vi "Lock In Time Trace.vi"() -> ()   [LabVIEW 2011]
panel:
  in  "VISA session (for class)":refnum<visa-resource-name>
  in  "Display Type":u16(ring) items=["X %", "Y %", "X Calibrated", "Y Calibrated", "Mag %", "Mag Calibrated", "Phase Degrees", "Ratio", "Log Ratio", "ADC 1", "ADC 2", "ADC 3", "ADC 4", "Noise %", "Noise Calibrated", "Ref Frequency", "Equation 1", "Equation 2"]
  out "XY Graph":cluster{"Y":dbl[], "Y":dbl[]}[](graph)
  in  "Time Target (s)":dbl=1.0
  in  "stop":bool
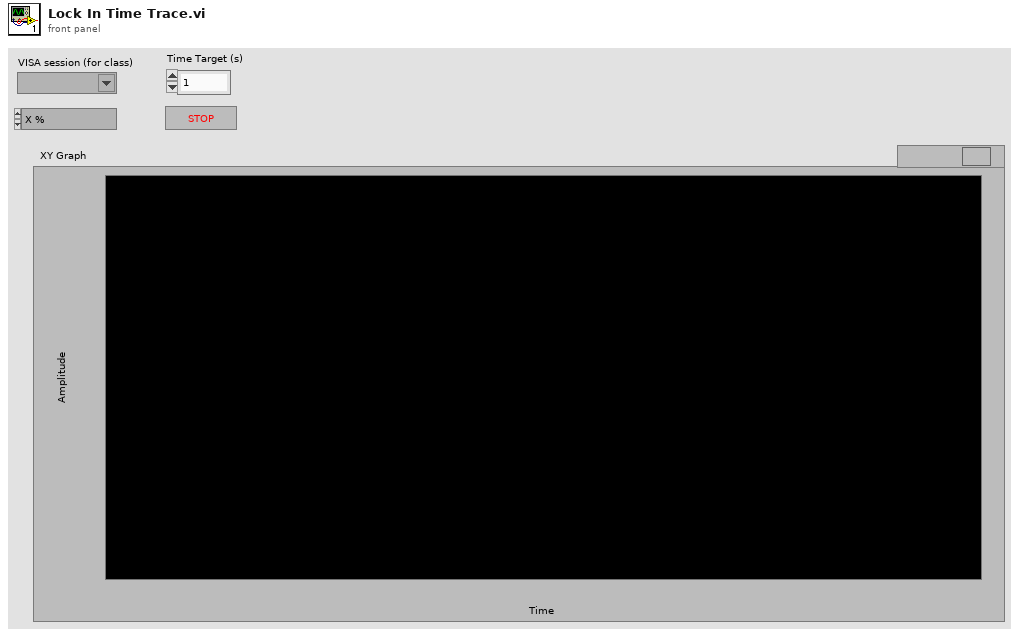
[diagram p1: front panel]
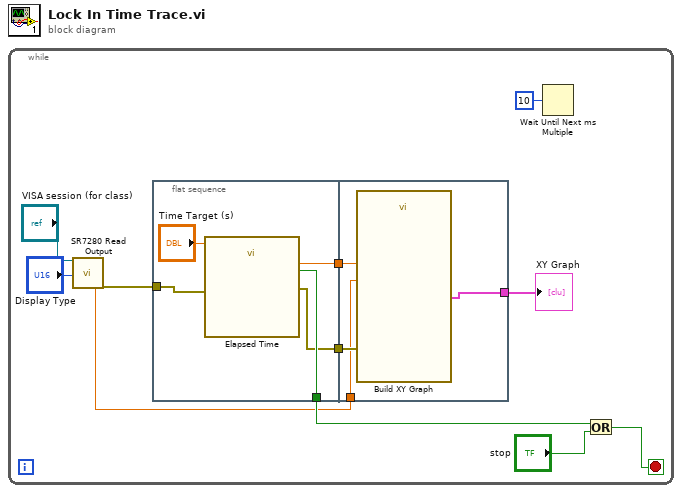
[diagram p0: block diagram]
diagram:
  n1 = while {
    stop <- w8 stop-if-true
    n2 = call "SR7280 Read Output.vi"("VISA session (for class)"="VISA session (for class)", "Display Type"="Display Type") -> ("Display"=w3:dbl, "error out"=w11:errorcluster)  [unwired: 9 in, 7 out]
    n3 = flat-sequence {
      tunnel: w11 -> [w16]
      tunnel: [w14] -> w10
      tunnel: [w13] -> w7
      tunnel: [w12] -> w6
      tunnel: w7 -> [w20]
      tunnel: w6 -> [w19]
      tunnel: [w18] -> w5
      tunnel: w3 -> [w17]
      frame #0 {
        n4 = call "Elapsed Time"("Time Target (s)"="Time Target (s)", "error in (no error)"=w16) -> ("Elapsed Time (s)"=w13:dbl, "Time has Elapsed"=w14:bool, "error out"=w12:errorcluster)  [unwired: 10 in, 5 out]
      }
      frame #1 {
        n5 = call "Build XY Graph"("error in (no error)"=w19, "Y Input"=w17, "X Input"=w20) -> ("XY Graph"=w18:cluster{"Y":dbl[], "Y":dbl[]}[])  [unwired: 2 in, 6 out]
      }
    }
    n6 = Wait Until Next ms Multiple(millisecond multiple=u32 10) -> ()  [unwired: 1 out]
    n7 = Or(x=w10, y="stop") -> (x .or. y?=w8:bool)
    "XY Graph" <- w5
  }
